vi "Add Default Enum.vi"(6 "Hdr Name":T1, 8 "error in (no error)":errorcluster, 9 "Enum Values":u16[](array[numeric]), 11 "Frequency in":refnum<class "Frequency.lvclass">) -> (0 "error out":errorcluster, 3 "Frequency out":refnum<class "Frequency.lvclass">)   [LabVIEW 2018, in "Measurement Channels.lvlib" / "Frequency.lvclass"]
uses:
  Frequency.lvclass
  Common/Controls/HeaderNames.ctl
  Frequency.lvclass/Frequency.ctl
  Class Voltage/Voltage.lvclass
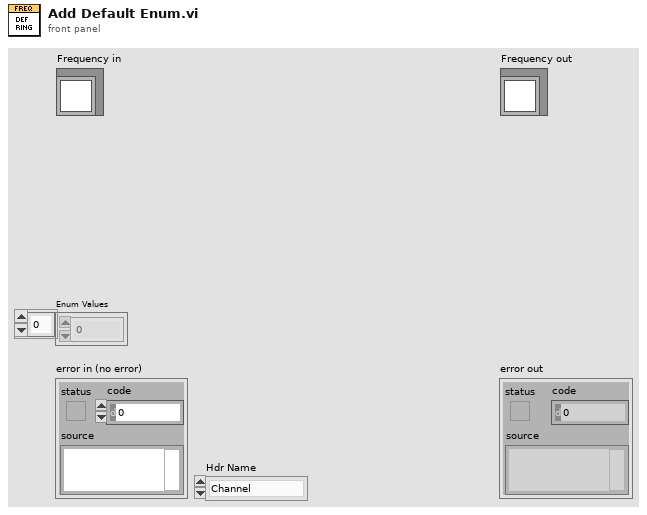
[diagram p1: front panel]
types:
  T1 = typedef "HeaderNames.ctl" = enum16{"Channel", "Device", "Spacer", "Description", "MB", "Range", "Terminal", "Coupling", "Thresh (V)", "Pulse/Rev", "Slope", "Min EU", "Min RPM", "mV/EU", "Iex", "Temp Units", "Type", "CJC Src", "CJC Val", "Ro", "Wire Cfg", "Strain Mode", "Vex", "Bridge Type", "GF", "Gauge Res", "Poisson", "Lead Res", "Init Strain", "GAF", "Scale", "Offset", "Unit (EU)", "dB?", "dB Ref", "Cal Mag", "Cal Units", "Max Temp", "Min Temp", "Max Strain", "Min Strain"}
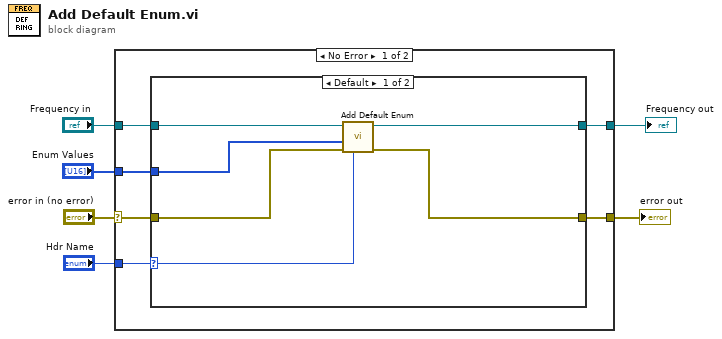
[diagram p0: block diagram]
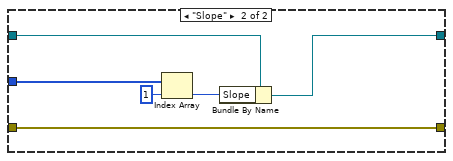
[diagram p2: hidden frame]
diagram:
  n1 = case shown="No Error" "error in (no error)" {
    selector: "error in (no error)" -> [w9 w26]
    tunnel: "Frequency in" -> [w12 w25]
    tunnel: [w11 w25] -> w5
    tunnel: "Hdr Name" -> [w10 _]
    tunnel: "Enum Values" -> [w8 _]
    tunnel: [w7 w26] -> w1
    frame No Error {
      n2 = case shown="Default" w10 {
        selector: w10 -> [w13 _]
        tunnel: w12 -> [w18 w24]
        tunnel: [w17 w23] -> w11
        tunnel: w9 -> [w16 w22]
        tunnel: w8 -> [w15 w20]
        tunnel: [w14 w22] -> w7
        frame Default {
          n3 = call-parent "Add Default Enum.vi"("Hdr Name"=w13, "error in (no error)"=w16, "Enum Values"=w15, "Voltage in"=w18) -> ("error out"=w14:errorcluster, "Voltage out"=w17:refnum<class "Frequency.lvclass">)  [unwired: 6 in]
        }
        frame "Slope" {
          n4 = Index Array(array=w20, index=1) -> (element=w19:u16)
          n5 = Bundle By Name(cluster=w24, "Slope"=w19) -> (w23:refnum<class "Frequency.lvclass">)
        }
      }
    }
    frame Error {
    }
  }
  "error out" <- w1
  "Frequency out" <- w5
